vi "Is prime-v1.vi"(8 "error in (no error)":errorcluster, 11 "x":i32) -> (0 "error out":errorcluster, 2 "T = x is prime":bool, 3 "First factor":i32)   [LabVIEW 2021, in "Numeric Utilities.lvlib"]
uses:
  Numeric Utilities.lvlib
panel:
  # "Development\ncontrols/indicators useful for development and testing, but which are not outputs of the VI"
  # "Input\nInputs to the VI"
  # "Output\nOutputs of the VI"
  # "Description\n\nBlank VI with error handling case. \n\nSummarize the use of this VI in this space."
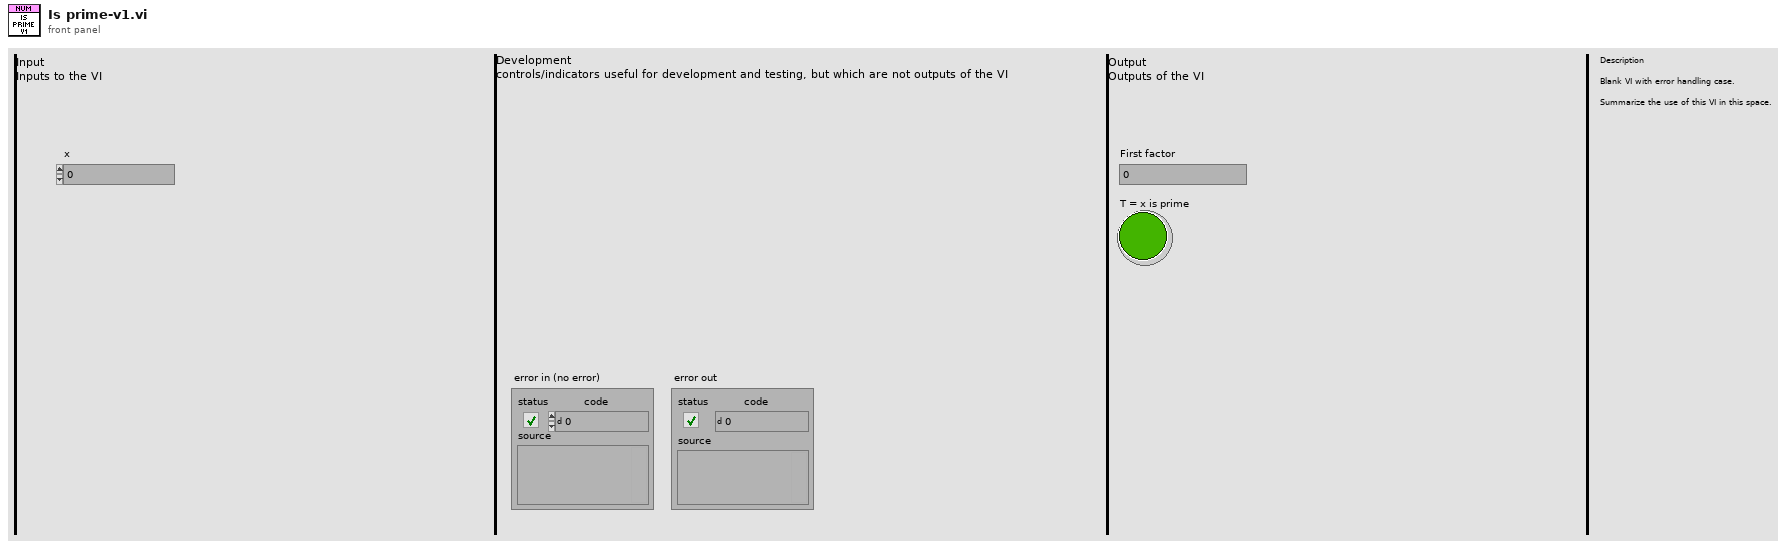
[diagram p1: front panel]
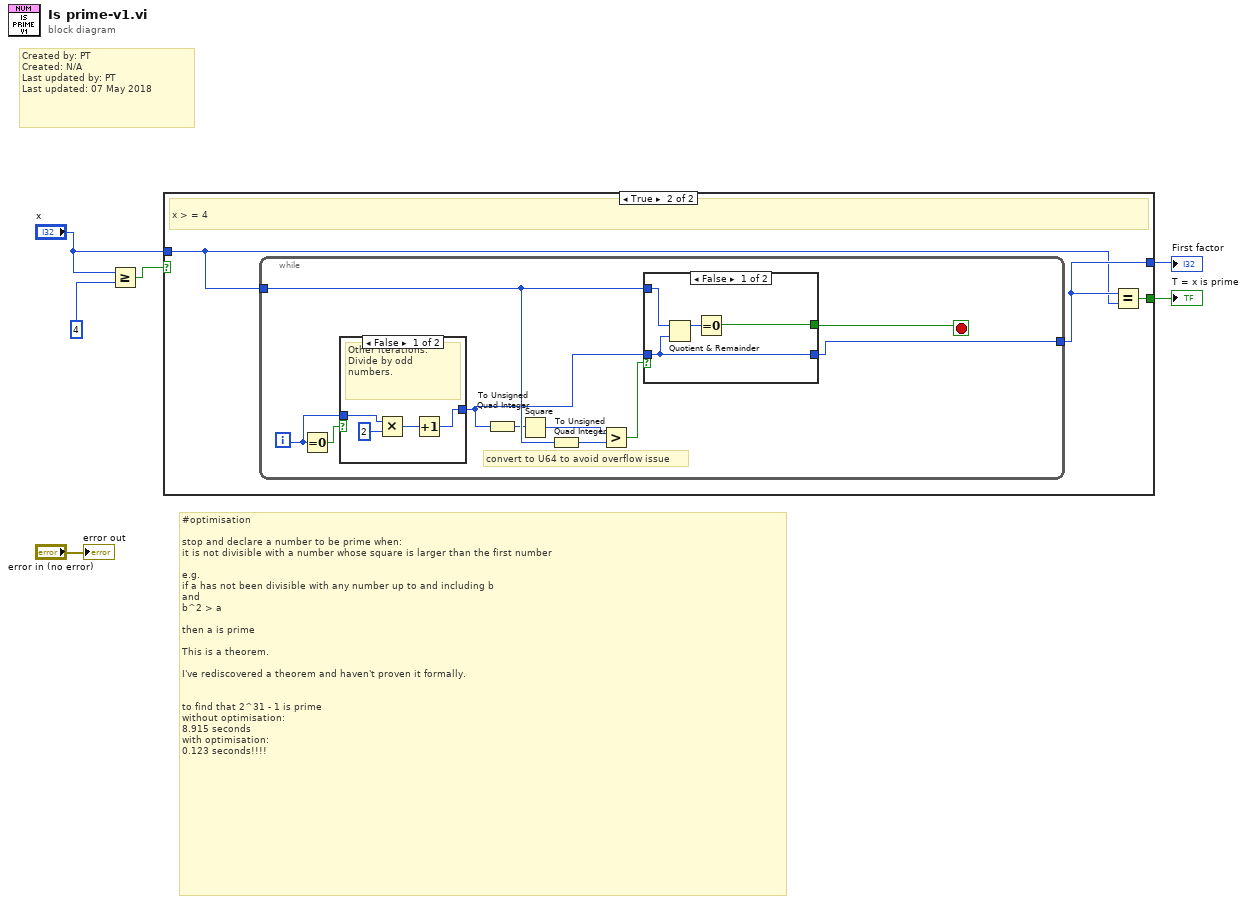
[diagram p0: block diagram]
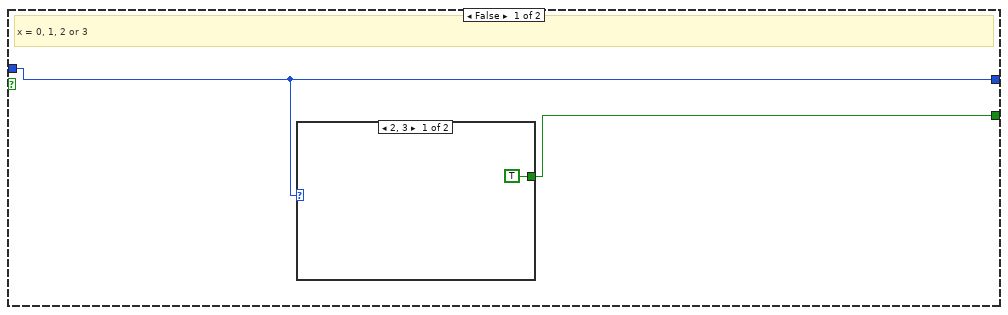
[diagram p2: hidden frame]
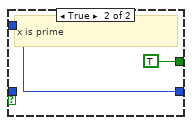
[diagram p4: hidden frame]
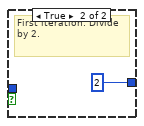
[diagram p5: hidden frame]
diagram:
  # "Created by: PT\nCreated: N/A\nLast updated by: PT\nLast updated: 07 May 2018"
  # "#optimisation\n\nstop and declare a number to be prime when:\nit is not divisible with a number whose square is larger than the first number\n\ne.g.\nif a has not been divisible with any number up to and including b\nand\nb^2 > a\n\nthen a is prime\n\nThis is a theorem.\n\nI've rediscovered a theorem and haven't proven it formally.\n\n\nto find that 2^31 - 1 is prime\nwithout optimisation:\n8.915 seconds\nwith optimisation:\n0.123 seconds!!!!"
  n1 = Greater Or Equal?(x="x", y=4) -> (x >= y?=w2:bool)
  n2 = case shown="True" w2 {
    tunnel: [w8 w12] -> w4
    tunnel: "x" -> [w8 w11]
    tunnel: [w7 w10] -> w1
    frame False {
      # "x = 0, 1, 2 or 3"
      n3 = case shown="2, 3" w8 {
        tunnel: [TRUE _] -> w7
        frame 2, 3 {
        }
        frame 0, 1, Default {
        }
      }
    }
    frame True {
      # "x > = 4"
      n4 = while {
        tunnel: w11 -> [w18]
        tunnel: [w15] -> w12
        i -> [w20]
        stop <- w22 stop-if-true
        # "convert to U64 to avoid overflow issue"
        n5 = Equal To 0?(x=w20) -> (x = 0?=w21:bool)
        n6 = case shown="False" w21 {
          tunnel: [w29 2] -> w16
          tunnel: w20 -> [w32 _]
          frame False {
            # "Other iterations. Divide by odd numbers."
            n7 = Multiply(x=w32, y=2) -> (x*y=w30:i32)
            n8 = Increment(x=w30) -> (x+1=w29:i32)
          }
          frame True {
            # "First iteration. Divide by 2."
          }
        }
        n9 = To Unsigned Quad Integer(1:w16) -> (0:w14:u64)
        n10 = Square(x=w14) -> (x^2=w19:u64)
        n11 = To Unsigned Quad Integer(1:w18) -> (0:w13:u64)
        n12 = Greater?(x=w19, y=w13) -> (0:w17:bool)
        n13 = case shown="False" w17 {
          tunnel: [w25 TRUE] -> w22
          tunnel: w16 -> [w23 _]
          tunnel: w18 -> [w24 w28]
          tunnel: [w23 w28] -> w15
          frame False {
            n14 = Quotient & Remainder(x=w24, y=w23) -> (x-y*floor(x/y)=w26:i32)  [unwired: 1 out]
            n15 = Equal To 0?(x=w26) -> (x = 0?=w25:bool)
          }
          frame True {
            # "x is prime"
          }
        }
      }
      n16 = Equal?(x=w12, y=w11) -> (x = y?=w10:bool)
    }
  }
  "First factor" <- w4
  "T = x is prime" <- w1
  "error out" <- "error in (no error)"
